vi "五子棋.vi"() -> ()   [LabVIEW 2019, in "五子棋.lvlib"]
uses:
  Status.ctl
  SetPiece.ctl
panel:
  out "狀態":string
  out "黑子":T1[][](array[typedef])
  out "白子":T2[][](array[typedef])
  # "五子棋程式-1（練習Event搭配State Machine的結構)\n1. 練習如何建立棋盤、黑子、白子；\n2. 按下「半黑白」可產生上下各一半的棋子，再按一次清除；\n3. 在滑鼠按下處，產生黑子；再按一次可以消除；"
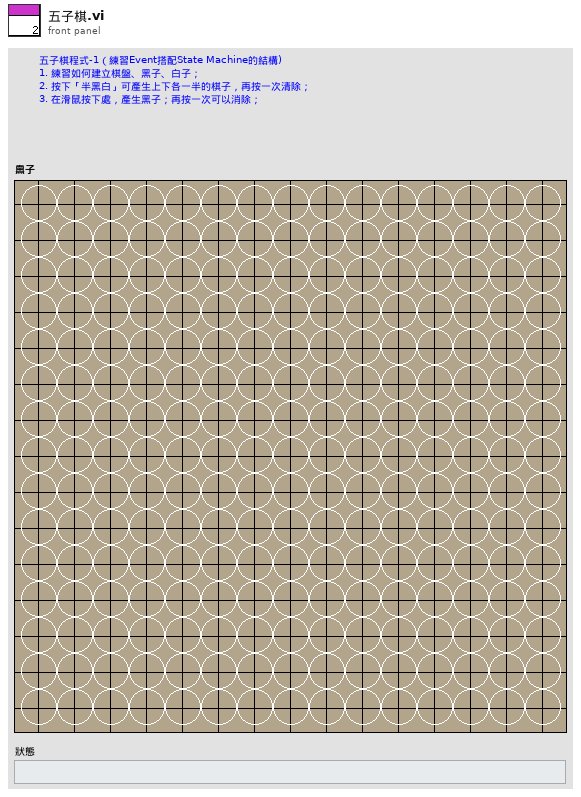
[diagram p1: front panel]
types:
  T1 = typedef "五子棋.lvlib/黑子.ctl" = bool
  T2 = typedef "五子棋.lvlib/白子.ctl" = bool
  T3 = typedef "五子棋.lvlib/Status.ctl" = enum16{"Idle", "Initialize", "Set Piece", "Check Win", "Computer Play"}
  T4 = typedef "LVPositionTypeDef.ctl" = cluster{"Left":i32, "Top":i32}
  T5 = typedef "LVBoundsTypeDef.ctl" = cluster{"Width":u32, "Height":u32}
  T6 = typedef "五子棋.lvlib/SetPiece.ctl" = cluster{"Row":i32, "Col":i32, "Black?":bool}
  T7 = typedef "LVPoint32TypeDef.ctl" = cluster{"Horizontal":i32, "Vertical":i32}
  T8 = typedef "Event 2-上課練習.lvlib/黑子.ctl" = bool
  T9 = typedef "Event 2-上課練習.lvlib/白子.ctl" = bool
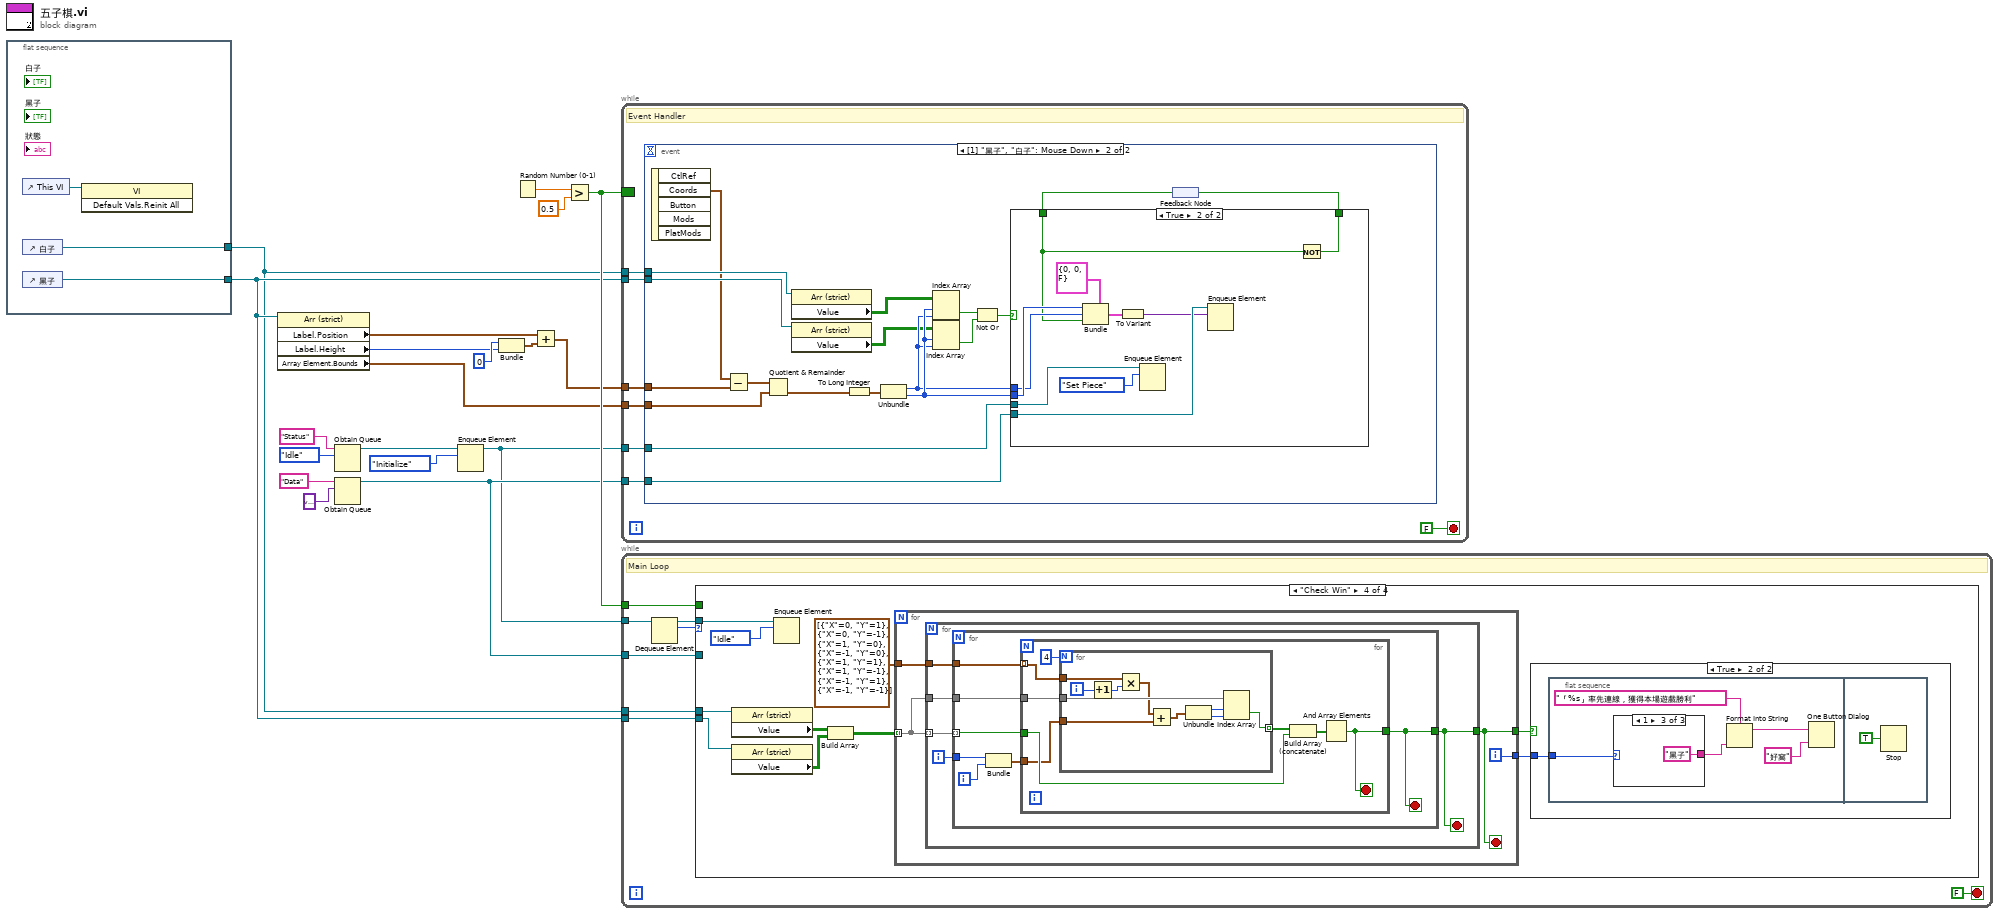
[diagram p0: block diagram]
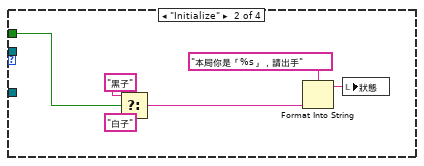
[diagram p3: hidden frame]
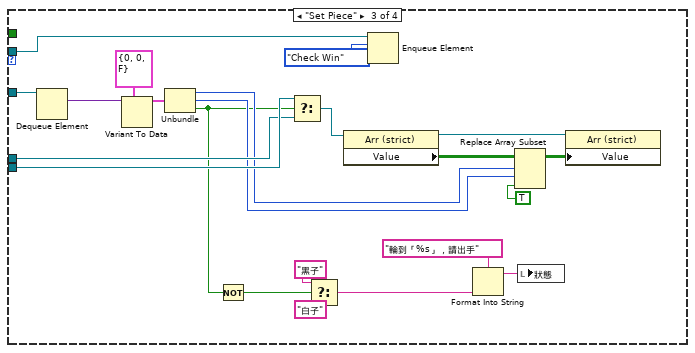
[diagram p4: hidden frame]
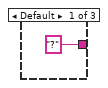
[diagram p6: hidden frame]
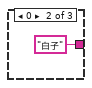
[diagram p7: hidden frame]
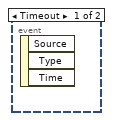
[diagram p8: hidden frame]
diagram:
  n1 = flat-sequence {
    tunnel: [w21] -> w13
    tunnel: [w20] -> w12
    frame #0 {
      n2 = control-ref of="This VI"() -> (w22:refnum<vi>)
      n3 = control-ref of="白子"() -> (w20:refnum<vi>)
      n4 = control-ref of="黑子"() -> (w21:refnum<vi>)
      n5 = invoke class="VI" method="Default Vals.Reinit All"(reference=w22) -> ()  [unwired: 2 in, 3 out]
    }
  }
  n6 = property class="Arr (strict)"(reference=w13) -> ("Label.Position"=w11:T4, "Label.Height"=w7:u32, "Array Element.Bounds"=w6:T5)  [unwired: 1 in, 2 out]
  n7 = Obtain Queue(name (unnamed)="Status", element data type=Status."Idle" ("Status")) -> (queue out=w3:refnum<queue>)  [unwired: 3 in, 2 out]
  n8 = Obtain Queue(name (unnamed)="Data", element data type=variant) -> (queue out=w14:refnum<queue>)  [unwired: 3 in, 2 out]
  n9 = Enqueue Element(queue=w3, element=Status."Initialize" ("Status")) -> (queue out=w2:refnum<queue>)  [unwired: 2 in, 2 out]
  n10 = Bundle(0, "Label.Height"=w7) -> (w10:cluster{i32, "Label.Height":u32})  [unwired: 1 in]
  n11 = Random Number (0-1)() -> (number: 0 to 1=w5:dbl)
  n12 = Add(x=w11, y=w10) -> (x+y=w9:cluster{i32, u32})
  n13 = Greater?(x=w5, y=0.5) -> (0:w19:bool)
  n14 = while {
    tunnel: w13 -> [w28]
    tunnel: w12 -> [w27]
    tunnel: w6 -> [w26]
    tunnel: w2 -> [w25]
    tunnel: w14 -> [w24]
    tunnel: w9 -> [w23]
    border: w19 -> [_]
    stop <- FALSE stop-if-true
    # "Event Handler"
    n15 = event shown="[1] \"黑子\", \"白子\": Mouse Down" {
      selector: _ -> [_ _]
      dyn-events: _ -> [_ _]
      timeout: _ -> [_ _]
      tunnel: w28 -> [_ w46]
      tunnel: w27 -> [_ w47]
      tunnel: w26 -> [_ w33]
      tunnel: w25 -> [_ w38]
      tunnel: w24 -> [_ w37]
      tunnel: w23 -> [_ w35]
      event Timeout {
        n16 = event-data() -> ()  [unwired: 1 in, 3 out]
      }
      event "黑子", "白子": Mouse Down {
        n17 = event-data() -> ("Coords"=w36:T7)  [unwired: 1 in, 4 out]
        n18 = Subtract(x=w36, y=w35) -> (x-y=w34:cluster{i32, u32})
        n19 = Quotient & Remainder(x=w34, y=w33) -> (floor(x/y)=w32:T5)  [unwired: 1 out]
        n20 = property class="Arr (strict)"(reference=w47) -> ("Value"=w45:T8[][])  [unwired: 1 in, 2 out]
        n21 = property class="Arr (strict)"(reference=w46) -> ("Value"=w42:T8[][])  [unwired: 1 in, 2 out]
        n22 = To Long Integer(number=w32) -> (32bit integer=w48:cluster{"Width":i32, "Height":i32})
        n23 = Unbundle(w48) -> ("Width"=w43:i32, "Height"=w44:i32)
        n24 = Index Array(array=w45, index (row)=w44, index (col)=w43) -> (element=w41:T8)
        n25 = Index Array(array=w42, index (row)=w44, index (col)=w43) -> (element=w40:T8)
        n26 = Not Or(1:w40, 2:w41) -> (0:w39:T8)
        n27 = feedback #1() -> (w30:bool)
        n28 = case shown="True" w39 {
          tunnel: w44 -> [_ w56]
          tunnel: w43 -> [_ w55]
          tunnel: w38 -> [_ w59]
          tunnel: w37 -> [_ w54]
          tunnel: [w49 w51] -> w31
          tunnel: w30 -> [w49 w50]
          frame False {
          }
          frame True {
            n29 = Bundle(cluster=T6 {"Row"=0, "Col"=0, "Black?"=FALSE}, "Row"=w56, "Col"=w55, "Black?"=w50) -> (w53:T6)
            n30 = To Variant(anything=w53) -> (Variant=w52:variant)
            n31 = Enqueue Element(queue=w59, element=Status."Set Piece") -> ()  [unwired: 2 in, 3 out]
            n32 = Enqueue Element(queue=w54, element=w52) -> ()  [unwired: 2 in, 3 out]
            n33 = Not(x=w50) -> (.not. x?=w51:bool)
          }
        }
        n34 = feedback-in #1(w31) -> ()
      }
    }
  }
  n35 = while {
    tunnel: w2 -> [w67]
    tunnel: w14 -> [w61]
    tunnel: w13 -> [w65]
    tunnel: w12 -> [w64]
    tunnel: w19 -> [w60]
    stop <- FALSE stop-if-true
    # "Main Loop"
    n36 = Dequeue Element(queue=w67) -> (queue out=w62:refnum<queue>, element=w66:T3)  [unwired: 2 in, 2 out]
    n37 = case shown="\"Check Win\"" w66 {
      tunnel: w65 -> [_ _ w88 w102]
      tunnel: w64 -> [_ _ w87 w103]
      tunnel: w62 -> [_ _ w84 w104]
      tunnel: w61 -> [_ _ w82 _]
      tunnel: w60 -> [_ w73 _ _]
      frame "Idle", Default {
      }
      frame "Initialize" {
        n38 = Select(t="黑子", s=w73, f="白子") -> (s? t:f=w69:string)
        n39 = Format Into String(format string="本局你是「%s」，請出手", w69) -> (resulting string=w68:string)  [unwired: 2 in, 1 out]
        n40 = local write "狀態"(w68) -> ()
      }
      frame "Set Piece" {
        n41 = Dequeue Element(queue=w82) -> (element=w81:variant)  [unwired: 2 in, 3 out]
        n42 = Variant To Data(type=T6 {"Row"=0, "Col"=0, "Black?"=FALSE}, Variant=w81) -> (data=w89:T6)  [unwired: 1 in, 1 out]
        n43 = Unbundle(w89) -> ("Row"=w86:i32, "Col"=w85:i32, "Black?"=w76:bool)
        n44 = Not(x=w76) -> (.not. x?=w75:bool)
        n45 = Select(t=w88, s=w76, f=w87) -> (s? t:f=w92:refnum<vi>)
        n46 = Select(t="黑子", s=w75, f="白子") -> (s? t:f=w77:string)
        n47 = property class="Arr (strict)"(reference=w92) -> (reference out=w90:refnum<vi>, "Value"=w91:T8[][])  [unwired: 1 in, 1 out]
        n48 = Enqueue Element(queue=w84, element=Status."Check Win") -> ()  [unwired: 2 in, 3 out]
        n49 = Format Into String(format string="輪到「%s」，請出手", w77) -> (resulting string=w74:string)  [unwired: 2 in, 1 out]
        n50 = Replace Array Subset(array=w91, new element=T1 TRUE ("new element/subarray"), index (row)=w86, index (col)=w85) -> (w93:T8[][])
        n51 = local write "狀態"(w74) -> ()
        n52 = property class="Arr (strict)"(reference=w90, "Value"=w93) -> ()  [unwired: 1 in, 2 out]
      }
      frame "Check Win" {
        n53 = property class="Arr (strict)"(reference=w103) -> ("Value"=w101:T9[][])  [unwired: 1 in, 2 out]
        n54 = property class="Arr (strict)"(reference=w102) -> ("Value"=w100:T9[][])  [unwired: 1 in, 2 out]
        n55 = Enqueue Element(queue=w104, element=Status."Idle") -> ()  [unwired: 2 in, 3 out]
        n56 = Build Array(w101, w100) -> (w99:T9[][][])
        n57 = for {
          tunnel: w99 -> [w118] mode=indexing
          tunnel: cluster{"X":i32, "Y":i32}[] [{"X"=0, "Y"=1}, {"X"=0, "Y"=-1}, {"X"=1, "Y"=0}, {"X"=-1, "Y"=0}, {"X"=1, "Y"=1}, {"X"=1, "Y"=-1}, {"X"=-1, "Y"=1}, {"X"=-1, "Y"=-1}] -> [w119]
          tunnel: [w117] -> w97
          tunnel: [w116] -> w96
          i -> [w116]
          stop <- w117 stop-if-true
          n58 = for {
            tunnel: w118 -> [w123] mode=indexing
            tunnel: w119 -> [w124]
            tunnel: w118 -> [w122]
            tunnel: [w121] -> w117
            i -> [w120]
            stop <- w121 stop-if-true
            n59 = for {
              tunnel: w123 -> [w131] mode=indexing
              tunnel: w124 -> [w130]
              tunnel: w122 -> [w129]
              tunnel: [w128] -> w121
              tunnel: w120 -> [w127]
              i -> [w126]
              stop <- w128 stop-if-true
              n60 = Bundle(w127, w126) -> (w125:cluster{i32, i32})  [unwired: 1 in]
              n61 = for {
                tunnel: w131 -> [w136]
                tunnel: w130 -> [w132] mode=indexing
                tunnel: w129 -> [w139]
                tunnel: [w134] -> w128
                tunnel: w125 -> [w133]
                stop <- w134 stop-if-true
                n62 = for {
                  N: 4 -> [_]
                  tunnel: w139 -> [w149]
                  tunnel: [w146] -> w137 mode=indexing
                  tunnel: w133 -> [w145]
                  tunnel: w132 -> [w142]
                  i -> [w143]
                  n63 = Increment(x=w143) -> (x+1=w141:i32)
                  n64 = Multiply(x=w142, y=w141) -> (x*y=w140:cluster{"X":i32, "Y":i32})
                  n65 = Add(x=w140, y=w145) -> (x+y=w144:cluster{i32, i32})
                  n66 = Unbundle(w144) -> (w148:i32, w147:i32)
                  n67 = Index Array(array=w149, index (row)=w148, index (col)=w147) -> (element=w146:T9)
                }
                n68 = Build Array (concatenate)(w137, w136) -> (w135:T9[])
                n69 = And Array Elements(Boolean array=w135) -> (logical AND=w134:bool)
              }
            }
          }
        }
        n70 = case shown="True" w97 {
          tunnel: w96 -> [_ w106]
          frame False {
          }
          frame True {
            n71 = flat-sequence {
              tunnel: w106 -> [w110]
              frame #0 {
                n72 = case shown="1" w110 {
                  tunnel: ["?" "白子" "黑子"] -> w109
                  frame Default {
                  }
                  frame 0 {
                  }
                  frame 1 {
                  }
                }
                n73 = Format Into String(format string="「%s」率先連線，獲得本場遊戲勝利", w109) -> (resulting string=w108:string)  [unwired: 2 in, 1 out]
                n74 = One Button Dialog(message=w108, button name ("OK")="好窩") -> ()  [unwired: 1 out]
              }
              frame #1 {
                n75 = Stop(stop? (T)=TRUE) -> ()
              }
            }
          }
        }
      }
    }
  }
